vi "Test Example Cluster 1 get some info.vi"() -> ()   [LabVIEW 2014]
panel:
  out "wire names":string[](array[string])
  out "terminals owners":string[](array[string])
  in  "vi path":path=path "C:/Users/lubo/Documents/LabView/LabVIEW-Universal-Transcriptor/Test/Examples For Parsing/Example Cluster 1.vi"
  in  "Error In":errorcluster
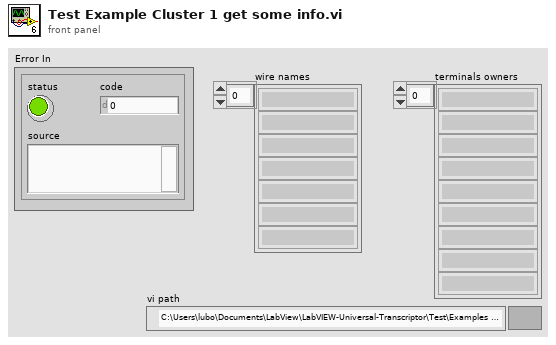
[diagram p1: front panel]
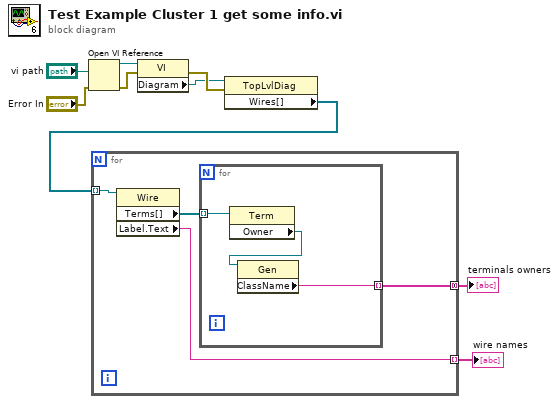
[diagram p0: block diagram]
diagram:
  n1 = Open VI Reference(vi path="vi path", error in (no error)="Error In") -> (vi reference=w8:refnum<vi>, error out=w7:errorcluster)  [unwired: 4 in]
  n2 = property class="VI"(reference=w8, error in=w7) -> (error out=w5:errorcluster, "Diagram"=w4:refnum<vi>)  [unwired: 1 out]
  n3 = property class="TopLvlDiag"(reference=w4, error in=w5) -> ("Wires[]"=w3:refnum<vi>[])  [unwired: 2 out]
  n4 = for {
    tunnel: w3 -> [w13] mode=indexing
    tunnel: [w11] -> w1 mode=indexing
    tunnel: [w10] -> w2 mode=concatenating
    n5 = property class="Wire"(reference=w13) -> ("Terms[]"=w12:refnum<vi>[], "Label.Text"=w11:string)  [unwired: 1 in, 2 out]
    n6 = for {
      tunnel: w12 -> [w16] mode=indexing
      tunnel: [w14] -> w10 mode=indexing
      n7 = property class="Term"(reference=w16) -> ("Owner"=w15:refnum<vi>)  [unwired: 1 in, 2 out]
      n8 = property class="Gen"(reference=w15) -> ("ClassName"=w14:string)  [unwired: 1 in, 2 out]
    }
  }
  "terminals owners" <- w2
  "wire names" <- w1
